vi "Loop Time- Seconds 03.vi"(9 "Loop Iteration":i32, 10 "Shift Registered Time In":u32, 11 "Shift Registered In":dbl) -> (1 "t":dbl, 2 "Shift Registered Time Out":u32, 3 "Shift Registered Out":dbl)   [LabVIEW 2018]
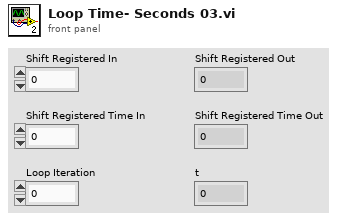
[diagram p1: front panel]
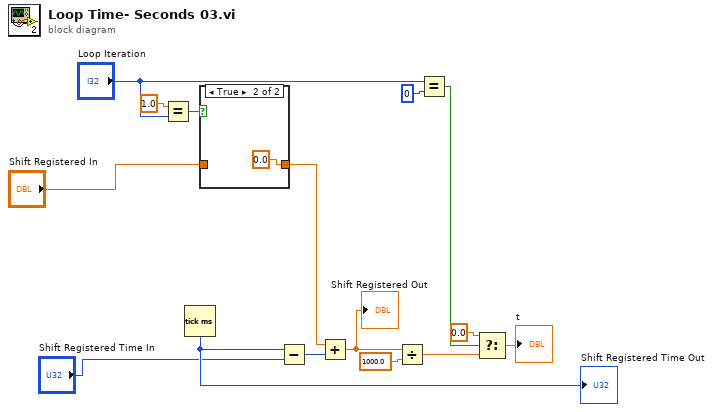
[diagram p0: block diagram]
diagram:
  n1 = Equal?(x=1.0, y="Loop Iteration") -> (x = y?=w4:bool)
  n2 = Tick Count (ms)() -> (millisecond timer value=w13:u32)
  "Shift Registered Time Out" <- w13
  n3 = case shown="True" w4 {
    tunnel: [w16 0.0] -> w6
    tunnel: "Shift Registered In" -> [w16 _]
    frame False {
    }
    frame True {
    }
  }
  n4 = Subtract(x=w13, y="Shift Registered Time In") -> (x-y=w7:u32)
  n5 = Add(x=w6, y=w7) -> (x+y=w14:dbl)
  "Shift Registered Out" <- w14
  n6 = Divide(x=w14, y=1000.0) -> (x/y=w8:dbl)
  n7 = Equal?(x="Loop Iteration", y=0) -> (x = y?=w11:bool)
  n8 = Select(t=0.0, s=w11, f=w8) -> (s? t:f=→"t":dbl)
